vi "niScope Initialize.vi"(0 "resource name":refnum<k15>="DAQ::1", 5 "id query":bool, 9 "reset device":bool=TRUE, 11 "error in":errorcluster) -> (4 "instrument handle":refnum<k15>, 15 "error out":errorcluster)   [LabVIEW 2013]
doc: "Performs the following initialization actions:\n\n--Creates a new IVI instrument driver session.\n\n-Opens a session to the device that you specify in the resource name parameter.\n\n-Queries the instrument ID and checks that it is valid for this instrument driver, if the id query parameter is set to TRUE.\n\n-Resets the instrument to a known state if the reset device parameter is set to TRUE; refer to niScope Reset for the default state of each digitizer.\n\n-Sends initialization commands to set the instrument to the state necessary for the operation of the instrument driver.\n\n-Returns an instrument handle that you use to identify the instrument in all subsequent instrument driver VI calls."
uses:
  niScope_32.dll
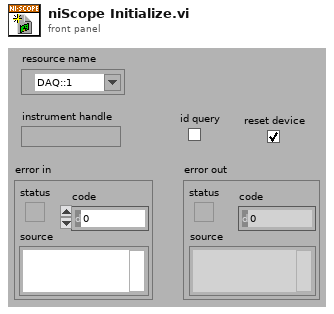
[diagram p1: front panel]
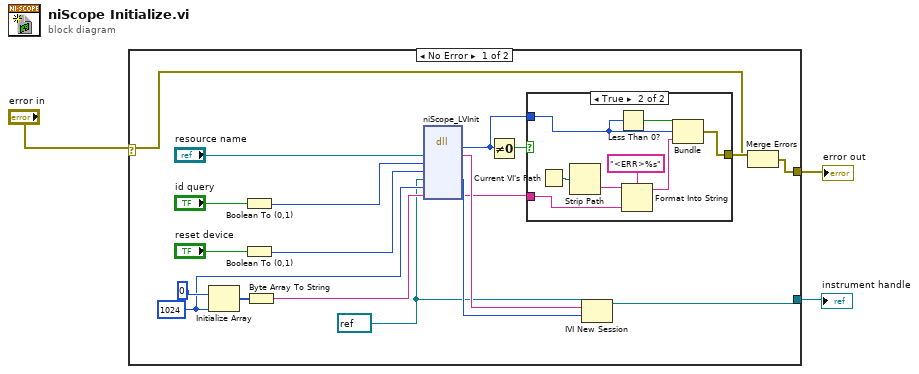
[diagram p0: block diagram]
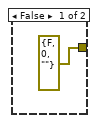
[diagram p2: hidden frame]
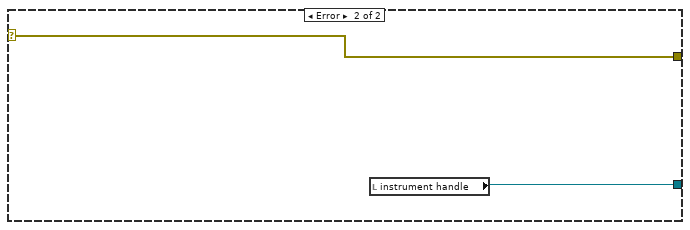
[diagram p3: hidden frame]
diagram:
  n1 = case shown="No Error" "error in" {
    selector: "error in" -> [w5 w32]
    tunnel: [w6 w32] -> w3
    tunnel: [w17 w33] -> w2
    frame No Error {
      w4 = refnum<k15> refnum
      w10 = 1024
      n2 = Initialize Array(0, w10) -> (w11:i32[])
      n3 = Boolean To (0,1)(Boolean="id query") -> (0, 1=w19:i16)
      n4 = Boolean To (0,1)(Boolean="reset device") -> (0, 1=w18:i16)
      n5 = Byte Array To String(unsigned byte array=w11) -> (string=w9:string)
      n6 = dll-call lib="niScope_*.*" fn="niScope_LVInit"("resourceName"="resource name", "IDQuery"=w19, "resetDevice"=w18, "instrument handle"=w4, "error buffer size"=w10, "error buffer"=w9) -> ("status"=w13:i32, "resourceName"=w16:string, "instrument handle"=w15:u32, "error buffer"=w8:string)  [unwired: 6 in, 2 out]
      n7 = Not Equal To 0?(x=w13) -> (x != 0?=w14:bool)
      n8 = case shown="True" w14 {
        tunnel: w8 -> [_ w31]
        tunnel: w13 -> [_ w26]
        tunnel: [cluster{bool, "status":i32, string} {FALSE, "status"=0, ""} w24] -> w7
        frame False {
        }
        frame True {
          n9 = Current VI's Path() -> (path=w29:path)
          n10 = Strip Path(path=w29) -> (name=w28:string)  [unwired: 1 out]
          n11 = Less Than 0?(x=w26) -> (x < 0?=w25:bool)
          n12 = Format Into String(format string="<ERR>%s", initial string=w28, w31) -> (resulting string=w27:string)  [unwired: 1 in, 1 out]
          n13 = Bundle(w25, "status"=w26, w27) -> (w24:cluster{bool, "status":i32, string})  [unwired: 1 in]
        }
      }
      n14 = IVI New Session(9:w15, 10:w16, 11:w4) -> (3:w17:refnum<k15>)
      n15 = Merge Errors(w5, w7) -> (w6:errorcluster)
    }
    frame Error {
      n16 = local read "instrument handle"() -> (w33:refnum<k15>)
    }
  }
  "error out" <- w3
  "instrument handle" <- w2
